vi "BuildNibble.vi"(7 "Read/Write Data":T1 {"Data" format="%.0x"}, 8 "error in (no error)":errorcluster, 9 "Number of Samples In":i32, 10 "Data Array In":u8[][](array[numeric]), 11 "RFFE_Data In":T2 {"Toggle (high to low)" items=["0", "1", "Z", "L", "H", "X", "T", "V"]; "X Array" items=["0", "1", "Z", "L", "H", "X", "T", "V"]; "Z Array" items=["0", "1", "Z", "L", "H", "X", "T", "V"]; "L Array" items=["0", "1", "Z", "L", "H", "X", "T", "V"]; "H Array" items=["0", "1", "Z", "L", "H", "X", "T", "V"]; "One Array" items=["0", "1", "Z", "L", "H", "X", "T", "V"]; "Zero Array" items=["0", "1", "Z", "L", "H", "X", "T", "V"]}) -> (0 "error out":errorcluster, 1 "Number of Samples Out":i32, 2 "Data Array Out":u8[][](array[numeric]), 3 "RFFE_Data Out":T2 {"Toggle (high to low)" items=["0", "1", "Z", "L", "H", "X", "T", "V"]; "X Array" items=["0", "1", "Z", "L", "H", "X", "T", "V"]; "Z Array" items=["0", "1", "Z", "L", "H", "X", "T", "V"]; "L Array" items=["0", "1", "Z", "L", "H", "X", "T", "V"]; "H Array" items=["0", "1", "Z", "L", "H", "X", "T", "V"]; "One Array" items=["0", "1", "Z", "L", "H", "X", "T", "V"]; "Zero Array" items=["0", "1", "Z", "L", "H", "X", "T", "V"]}, 4 "Parity Out":u8)   [LabVIEW 2013]
doc: "Adds a Start (S) or Repeated Start (Sr) condition to the I2C waveform. \n\nTiming parameters that affect this waveform segment's length are: <b>tSU;DAT</b> (Sr only), <b>tSU;STA</b> (Sr only), <b>tHD;STA </b>, and <b>tHD;DAT</b>"
uses:
  Ctrls/RFFE_Data.ctl
  Ctrls/ClockDataChannels.ctl
  Ctrls/Read_Write_Data.ctl
  Ctrls/BitStates.ctl
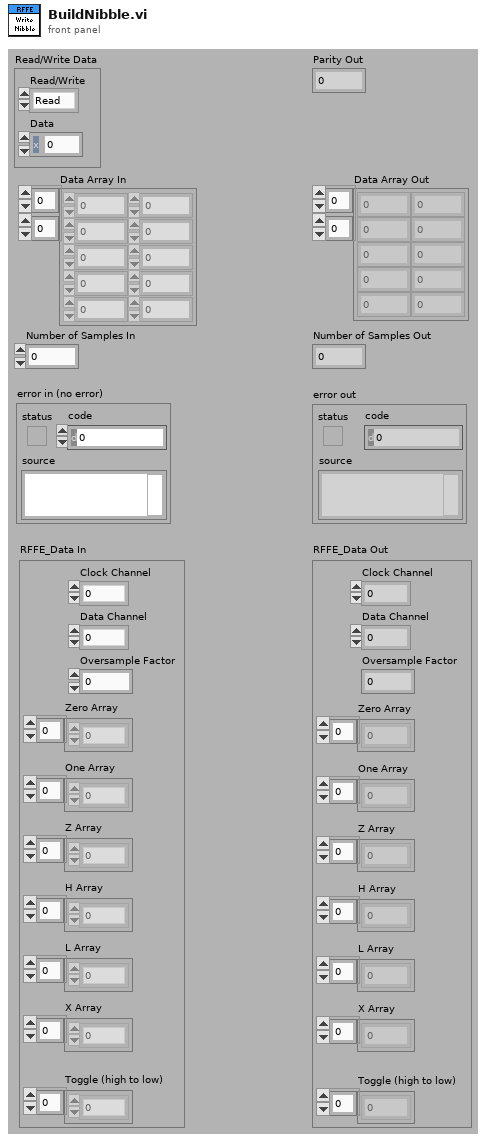
[diagram p1: front panel]
types:
  T1 = typedef "Read_Write_Data.ctl" = cluster{"Data":u8, "Read/Write":enum16{"Read", "Write"}}
  T2 = typedef "RFFE_Data.ctl" = cluster{"Clock Channel":T3, "Data Channel":T3, "Oversample Factor":u8, "Zero Array":u8[], "One Array":u8[], "Z Array ":u8[], "H Array":u8[], "L Array":u8[], "X Array":u8[], "Toggle (high to low)":u8[]}
  T3 = typedef "ClockDataChannels.ctl" = enum16{"0", "1"}
  T4 = typedef "BitStates.ctl" = enum16{"0", "1", "Z", "L", "H", "X", "Toggle"}
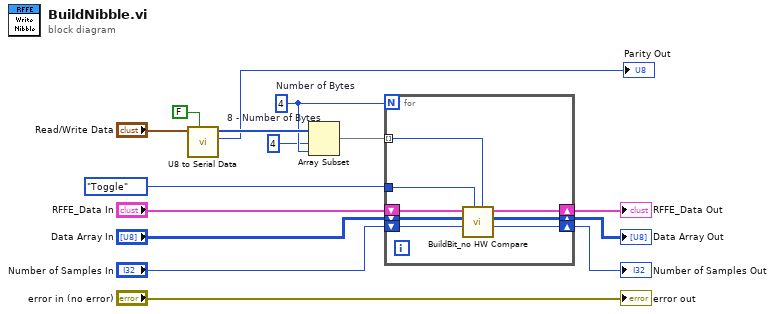
[diagram p0: block diagram]
diagram:
  w4 = 4  # 8 - Number of Bytes
  w5 = 4  # Number of Bytes
  n1 = call "U8 to Serial Data.vi"("Parity Bit?"=FALSE, "Read/Write Data"="Read/Write Data") -> ("Parity Out"=→"Parity Out":u8, "Data Values"=w8:T4[])  [unwired: 8 in]
  n2 = Array Subset(array=w8, index=w4, length=w5) -> (w6:T4[])
  n3 = for {
    N: w5 -> [_]
    tunnel: BitStates."Toggle" ("Data Value") -> [w20]
    shift-right: [w18] -> w13
    shift-left: "Data Array In" -> [w23]
    shift-right: [w17] -> w14
    shift-left: "RFFE_Data In" -> [w21]
    shift-right: [w19] -> w7
    shift-left: "Number of Samples In" -> [w22]
    tunnel: w6 -> [w16] mode=indexing
    n4 = call "BuildBit_no HW Compare.vi"("Data Value"=w16, "Clock Value"=w20, "Number of Samples In"=w22, "Data Array In"=w23, "RFFE_Data In"=w21) -> ("Number of Samples Out"=w19:i32, "Data Array Out"=w18:u8[][], "RFFE_Data Out"=w17:T2)  [unwired: 4 in]
  }
  "RFFE_Data Out" <- w14
  "Data Array Out" <- w13
  "Number of Samples Out" <- w7
  "error out" <- "error in (no error)"
